vi "Point to Item.vi"(8 "Error In":errorcluster, 10 "Coords":T1, 11 "reference":refnum<vi>) -> (0 "Error Out":errorcluster, 2 "Item":string)   [LabVIEW 2016]
uses:
  <vilib>/Utility/miscctls.llb/LVPoint32TypeDef.ctl
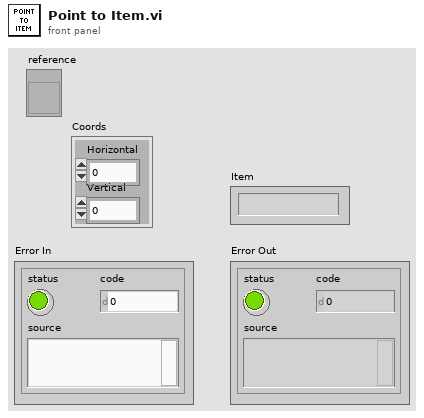
[diagram p1: front panel]
types:
  T1 = typedef "LVPoint32TypeDef.ctl" = cluster{"Horizontal":i32, "Vertical":i32}
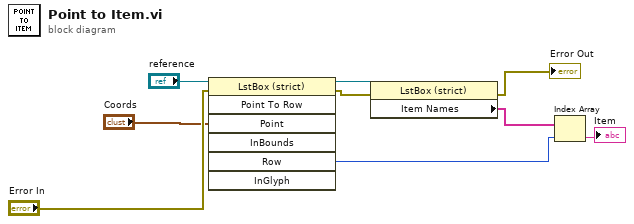
[diagram p0: block diagram]
diagram:
  n1 = invoke class="LstBox (strict)" method="Point To Row"(reference="reference", error in="Error In", "Point"="Coords") -> (reference out=w6:refnum<vi>, error out=w3:errorcluster, "Row"=w4:i32)  [unwired: 4 in, 4 out]
  n2 = property class="LstBox (strict)"(reference=w6, error in=w3) -> (error out=→"Error Out":errorcluster, "Item Names"=w5:string[])  [unwired: 1 out]
  n3 = Index Array(array=w5, index=w4) -> (element=→"Item":string)
